vi "Write Length.vi"(8 "error in (no error)":errorcluster, 10 "Length":u16, 11 "Update Filter Cycle Params MSG in":refnum<class "Update Filter Cycle Params MSG.lvclass">) -> (0 "error out":errorcluster, 3 "Update Filter Cycle Params MSG out":refnum<class "Update Filter Cycle Params MSG.lvclass">)   [LabVIEW 2014, in "Controller.lvlib" / "Update Filter Cycle Params MSG.lvclass"]
uses:
  Update Filter Cycle Params MSG.lvclass
  Update Filter Cycle Params MSG.lvclass/Update Filter Cycle Params MSG.ctl
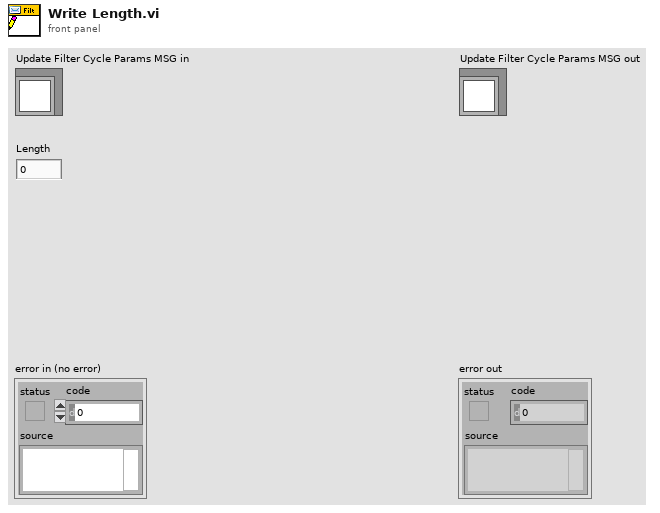
[diagram p1: front panel]
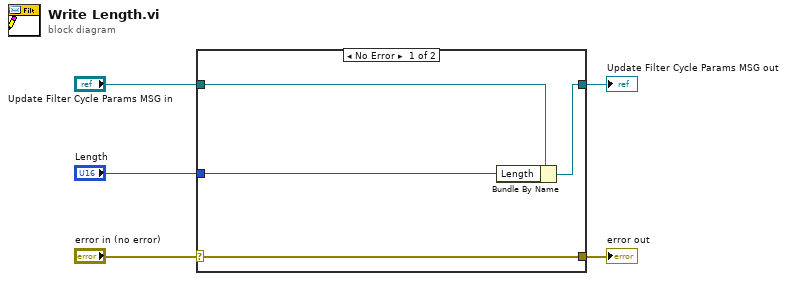
[diagram p0: block diagram]
diagram:
  n1 = case shown="No Error" "error in (no error)" {
    selector: "error in (no error)" -> [w9 w10]
    tunnel: [w9 w10] -> w4
    tunnel: [w7 w11] -> w2
    tunnel: "Update Filter Cycle Params MSG in" -> [w8 w11]
    tunnel: "Length" -> [w6 _]
    frame No Error {
      n2 = Bundle By Name(cluster=w8, "Length"=w6) -> (w7:refnum<class "Update Filter Cycle Params MSG.lvclass">)
    }
    frame Error {
    }
  }
  "error out" <- w4
  "Update Filter Cycle Params MSG out" <- w2
